vi "Dev List - Update DTRow.vi"(7 "Row Index":i32, 8 "error in (no error)":errorcluster, 9 "Dev Data Lookup Table in":variant, 10 "DataGridView in":refnum<class "DataGridView.lvclass">, 11 "Controller UI in":refnum<class "Controller UI.lvclass">) -> (0 "error out":errorcluster, 1 "Dev Data Lookup Table in out":variant, 2 "DataGridView out":refnum<class "DataGridView.lvclass">)   [LabVIEW 2016, in "Controller UI.lvlib" / "Controller UI.lvclass"]
uses:
  <userlib>/Common Components/Controller UI/Controller UI.lvclass
  C:/Program Files (x86)/National Instruments/LabVIEW 2016/vi.lib/ActorFramework/Actor/Actor.lvclass
  <userlib>/LabVIEWdotNetDataGrid/source/DataGridView/DataGridView.lvclass
  <userlib>/Common Components/Hardware/DevInfo/DevInfo.lvclass
  <userlib>/Common Components/Controller UI/Dev Variant Data.ctl
  <vilib>/ActorFramework/Actor/Actor.lvclass/Actor.ctl
  <userlib>/Common Components/Hardware/DevInfo/DevInfo.lvclass/DevInfo.ctl
  <userlib>/Common Components/Controller/Messages/Update a Dev Requested by UI Msg/Update a Dev Requested by UI Msg.lvclass/Update a Dev Requested by UI Msg.ctl
  <vilib>/ActorFramework/Message Enqueuer/Message Enqueuer.lvclass/Message Enqueuer.ctl
  <userlib>/Common Components/Hardware/DevInfo/Read GUID.vi
  <vilib>/ActorFramework/Message Enqueuer/Enqueue.vi
  <userlib>/Common Components/Controller/Messages/Update a Dev Requested by UI Msg/Update a Dev Requested by UI Msg.lvclass
  C:/Program Files (x86)/National Instruments/LabVIEW 2016/vi.lib/ActorFramework/Message/Message.lvclass
  <userlib>/LabVIEWdotNetDataGrid/source/DataGridView/Get DataRow (String).vi
  <vilib>/ActorFramework/Message Priority Queue/Priority Enqueue.vi
  <vilib>/ActorFramework/Actor/Actor.lvclass
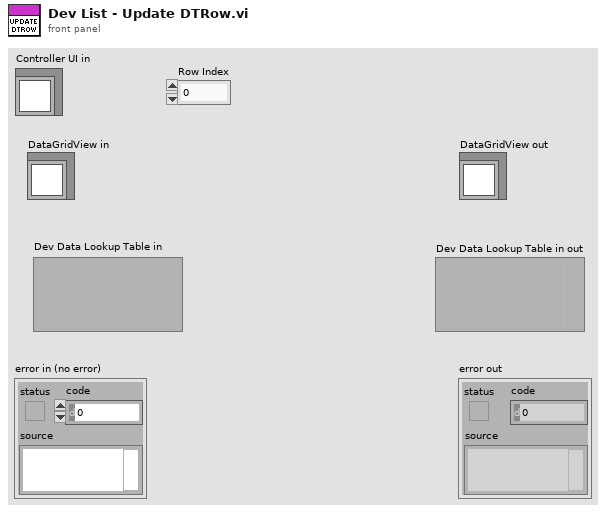
[diagram p1: front panel]
types:
  T1 = typedef "Controller UI.lvlib/Controller UI.lvclass/Dev Variant Data.ctl" = cluster{"Row Index":i32, "DevInfo Obj":refnum<class "DevInfo.lvclass">}
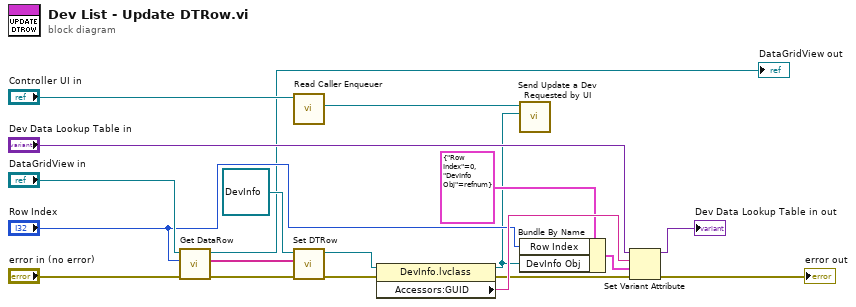
[diagram p0: block diagram]
diagram:
  n1 = call-poly <userlib>:"Get DataRow.vi"("error in (no error)"="error in (no error)", "index"="Row Index", "DataGridView in"="DataGridView in") -> ("error out"=w16:errorcluster, "Array"=w17:string[], "DataGridView out"=→"DataGridView out":refnum<class "DataGridView.lvclass">)  [unwired: 6 in]
  n2 = call <vilib>:"Read Caller Enqueuer.vi"("Actor"="Controller UI in") -> ("Caller Enqueuer"=w12:refnum<class "Message Enqueuer.lvclass">)  [unwired: 10 in]
  n3 = call <userlib>:"Set DTRow.vi"("error in (no error)"=w16, "Dev Row Elements"=w17, "DevInfo in"=refnum<class "DevInfo.lvclass"> refnum ("DevInfo")) -> ("error out"=w3:errorcluster, "DevInfo out"=w18:refnum<class "DevInfo.lvclass">)  [unwired: 7 in]
  n4 = property class="DevInfo.lvclass"(reference=w18, error in=w3) -> (reference out=w6:refnum<class "DevInfo.lvclass">, error out=w2:errorcluster, "Accessors:GUID"=w9:string)
  n5 = call <userlib>:"Send Update a Dev Requested by UI.vi"("DevInfo"=w6, "Message Enqueuer in"=w12) -> ()  [unwired: 8 in, 2 out]
  n6 = Bundle By Name(cluster=T1 {"Row Index"=0, "DevInfo Obj"=refnum} ("Dev Data Lookup Table"), "Row Index"="Row Index", "DevInfo Obj"=w6) -> (w5:T1)
  n7 = Set Variant Attribute(Variant="Dev Data Lookup Table in", name=w9, value=w5, error in=w2) -> (Variant out=→"Dev Data Lookup Table in out":variant, error out=→"error out":errorcluster)  [unwired: 1 out]
